vi "CheckInside.vi"(1 "rect":T1, 2 "Coords":T2) -> (0 "Inside?":bool)   [LabVIEW 2012]
uses:
  <vilib>/Utility/miscctls.llb/LVPoint32TypeDef.ctl
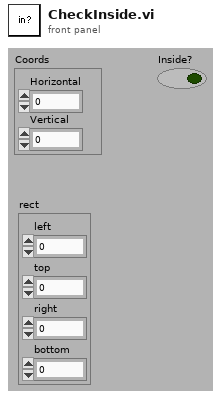
[diagram p1: front panel]
types:
  T1 = cluster{"left":i16, "top":i16, "right":i16, "bottom":i16}
  T2 = typedef "LVPoint32TypeDef.ctl" = cluster{"Horizontal":i32, "Vertical":i32}
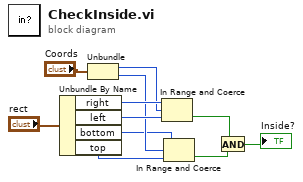
[diagram p0: block diagram]
diagram:
  n1 = Unbundle By Name("rect") -> ("right"=w9:i16, "left"=w7:i16, "bottom"=w4:i16, "top"=w3:i16)
  n2 = Unbundle("Coords") -> ("Horizontal"=w6:i32, "Vertical"=w5:i32)
  n3 = In Range and Coerce(upper limit=w9, x=w6, lower limit=w7) -> (In Range?=w10:bool)  [unwired: 1 out]
  n4 = In Range and Coerce(upper limit=w4, x=w5, lower limit=w3) -> (In Range?=w2:bool)  [unwired: 1 out]
  n5 = And(x=w10, y=w2) -> (x .and. y?=→"Inside?":bool)
